vi "waypoint_short.vi"(6 "semaphore":T1, 7 "Motor Adress":T2(ring)=enum."3", 8 "error in (no error)":errorcluster, 9 "steps":i32, 10 "Profile Number":i32=123456, 11 "VISA ressource in":refnum<visa-resource-name>="COM1") -> (0 "error out":errorcluster={"status"=FALSE, "code"=1073676294, "source"="VISA Read in write_read.vi"}, 1 "Delta Steps":i32, 2 "Log File":string, 3 "VISA ressource out":refnum<visa-resource-name>)   [LabVIEW 2013]
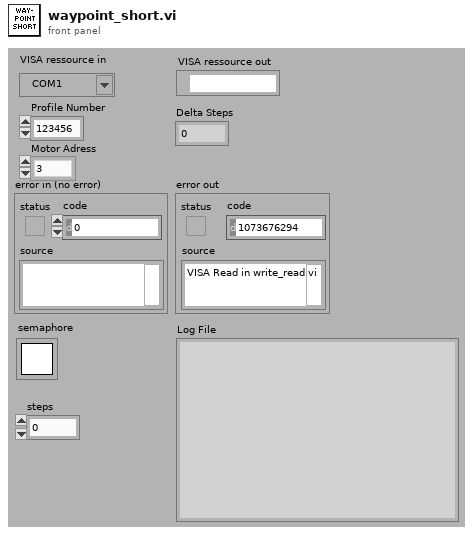
[diagram p1: front panel]
types:
  T1 = typedef "Semaphore RefNum" = refnum<k1>
  T2 = enum16{"All", "1", "2", "3", "4", "5", "6", "7", "8"}
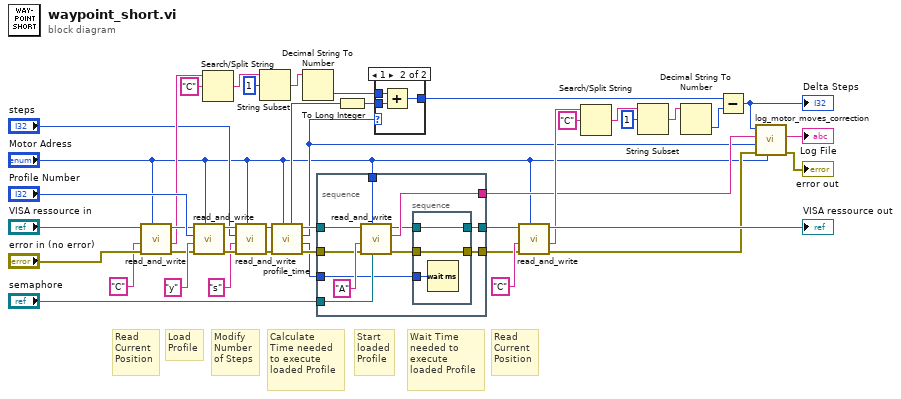
[diagram p0: block diagram]
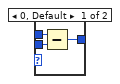
[diagram p2: hidden frame]
diagram:
  # "Modify\nNumber\nof Steps"
  # "Wait Time\nneeded to\nexecute\nloaded Profile"
  # "Read\nCurrent\nPosition"
  # "Start\nloaded\nProfile"
  # "Calculate\nTime needed\nto execute\nloaded Profile"
  # "Load\nProfile"
  # "Read\nCurrent\nPosition"
  n1 = call "read_and_write.vi"("Motor Adress"="Motor Adress", "error in (no error)"="error in (no error)", "Command"="C", "VISA ressource in"="VISA ressource in") -> ("error out"=w39:errorcluster, "Answer"=w31:string, "VISA ressource out"=w38:refnum<visa-resource-name>)  [unwired: 4 in, 1 out]
  n2 = call "read_and_write.vi"("Motor Adress"="Motor Adress", "error in (no error)"=w39, "Command"="y", "value"="Profile Number", "VISA ressource in"=w38) -> ("error out"=w9:errorcluster, "VISA ressource out"=w7:refnum<visa-resource-name>)  [unwired: 3 in, 2 out]
  n3 = Search/Split String(string=w31, search string/char (-)="C") -> (match + rest of string=w29:string)  [unwired: 1 in, 2 out]
  n4 = call "read_and_write.vi"("Motor Adress"="Motor Adress", "error in (no error)"=w9, "Command"="s", "value"="steps", "VISA ressource in"=w7) -> ("error out"=w8:errorcluster, "VISA ressource out"=w6:refnum<visa-resource-name>)  [unwired: 3 in, 2 out]
  n5 = String Subset(string=w29, offset (0)=1) -> (substring=w27:string)  [unwired: 1 in]
  n6 = call "profile_time.vi"("Motor Adress"="Motor Adress", "error in (no error)"=w8, "VISA ressource in"=w6) -> ("error out"=w34:errorcluster, "profile time (in ms)"=w16:u32, "direction"=w12:i32, "VISA ressource out"=w35:refnum<visa-resource-name>, "steps"=w19:u32)  [unwired: 4 in]
  n7 = Decimal String To Number(string=w27) -> (number=w20:i32)  [unwired: 2 in, 1 out]
  n8 = stacked-sequence {
    tunnel: w35 -> [w53]
    tunnel: w34 -> [w52]
    tunnel: [w51] -> w13
    tunnel: "semaphore" -> [w50]
    tunnel: "Motor Adress" -> [w49]
    tunnel: [w46] -> w2
    tunnel: [w45] -> w1
    tunnel: w16 -> [w44]
    frame #0 {
      n9 = call "read_and_write.vi"("semaphore"=w50, "Motor Adress"=w49, "error in (no error)"=w52, "Command"="A", "VISA ressource in"=w53) -> ("error out"=w47:errorcluster, "Log File (global)"=w51:string, "VISA ressource out"=w48:refnum<visa-resource-name>)  [unwired: 3 in, 1 out]
      n10 = stacked-sequence {
        tunnel: w48 -> [w56]
        tunnel: w47 -> [w57]
        tunnel: [w57] -> w45
        tunnel: [w56] -> w46
        tunnel: w44 -> [w55]
        frame #0 {
          n11 = Wait (ms)(milliseconds to wait=w55) -> ()  [unwired: 1 out]
        }
      }
    }
  }
  n12 = To Long Integer(number=w19) -> (32bit integer=w18:i32)
  n13 = case shown="1" w12 {
    tunnel: w20 -> [w60 w63]
    tunnel: w18 -> [w59 w62]
    tunnel: [w58 w61] -> w17
    frame 0, Default {
      n14 = Subtract(x=w60, y=w59) -> (x-y=w58:i32)
    }
    frame 1 {
      n15 = Add(x=w63, y=w62) -> (x+y=w61:i32)
    }
  }
  n16 = call "read_and_write.vi"("Motor Adress"="Motor Adress", "error in (no error)"=w1, "Command"="C", "VISA ressource in"=w2) -> ("error out"=w11:errorcluster, "Answer"=w22:string, "VISA ressource out"=→"VISA ressource out":refnum<visa-resource-name>)  [unwired: 4 in, 1 out]
  n17 = Search/Split String(string=w22, search string/char (-)="C") -> (match + rest of string=w24:string)  [unwired: 1 in, 2 out]
  n18 = String Subset(string=w24, offset (0)=1) -> (substring=w26:string)  [unwired: 1 in]
  n19 = Decimal String To Number(string=w26) -> (number=w21:i32)  [unwired: 2 in, 1 out]
  n20 = Subtract(x=w17, y=w21) -> (x-y=w15:i32)
  "Delta Steps" <- w15
  n21 = call "log_motor_moves_correction.vi"("Motor Adress"="Motor Adress", "error in"=w11, "Direction"=w12, "Log File IN"=w13, "Delta Steps"=w15) -> ("error out"=→"error out":errorcluster, "Log File OUT"=→"Log File":string)  [unwired: 5 in]
